vi "Execution Events Notifier.vi"(11 "Hierarchy (Auto)":string) -> (2 "created new?":bool, 3 "Events Notifier":refnum<notifier>)   [LabVIEW 2022 SP3, in "FlexBlocks Support.lvlib"]
uses:
  FlexBlocks Support.lvlib
  Block State.ctl
  Block Phase.ctl
  Block Status.ctl
  Block Status with Error.ctl
  Block Command.ctl
  Worker Block.ctl
  Worker Registration.ctl
  Execution Events.ctl
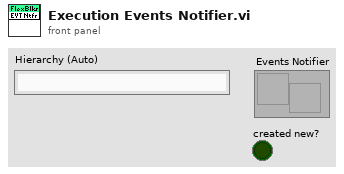
[diagram p1: front panel]
types:
  T1 = typedef "FlexBlocks Support.lvlib/Execution Events.ctl" = cluster{"Registration":refnum<user-event>, "Init":refnum<user-event>, "Run":refnum<user-event>, "Step":refnum<user-event>, "Stop":refnum<user-event>, "Close":refnum<user-event>, "Block Status":refnum<user-event>}
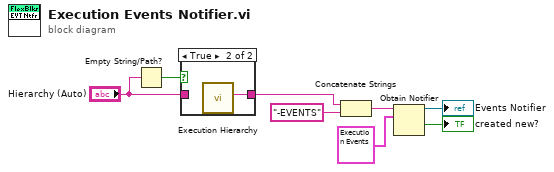
[diagram p0: block diagram]
diagram:
  n1 = Empty String/Path?(string/path="Hierarchy (Auto)") -> (empty?=w4:bool)
  n2 = case shown="True" w4 {
    tunnel: "Hierarchy (Auto)" -> [w9 _]
    tunnel: [w9 w10] -> w2
    frame False {
    }
    frame True {
      n3 = call "Execution Hierarchy.vi"() -> ("Top Level VI Name"=w10:string)  [unwired: 11 in]
    }
  }
  n4 = Concatenate Strings(w2, "-EVENTS" ("string")) -> (w7:string)
  n5 = Obtain Notifier(name (unnamed)=w7, notification data type=T1 {"Registration"=refnum, "Init"=refnum, "Run"=refnum, "Step"=refnum, "Stop"=refnum, "Close"=refnum, "Block Status"=refnum} ("Execution Events")) -> (notifier out=→"Events Notifier":refnum<notifier>, created new?=→"created new?":bool)  [unwired: 2 in, 1 out]
